vi "Test Array Data to Wave.vi"(7 "Datatype":string, 8 "error in (no error)":errorcluster, 9 "Data":variant, 10 "Dimension":string, 11 "Flag":string) -> (0 "error out":errorcluster)   [LabVIEW 2019, in "LV-Data.ITX.lvclass"]
uses:
  LV-Data.ITX.lvclass
  <vilib>/addons/_JKI Toolkits/Caraya/classes/Assert/Assert Equal Value_Variant.vi
  <vilib>/addons/_JKI Toolkits/Caraya/classes/Assert/Assert Almost Equal_Float.vi
  <vilib>/addons/_JKI Toolkits/Caraya/classes/Assert/Assert.lvclass
  <vilib>/addons/_JKI Toolkits/Caraya/classes/Test/Test.lvclass
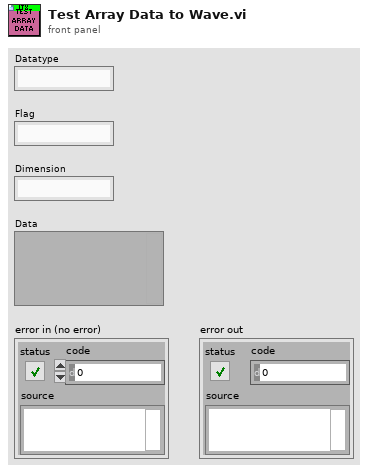
[diagram p1: front panel]
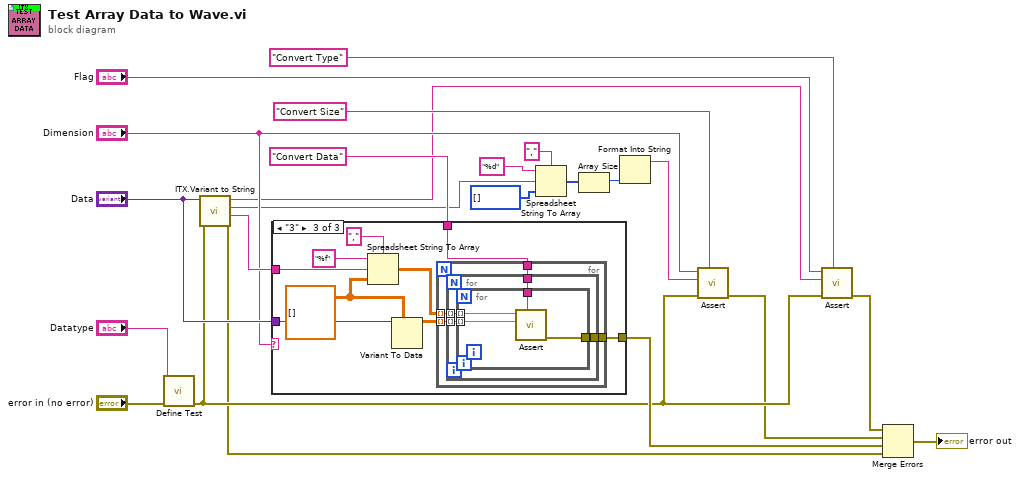
[diagram p0: block diagram]
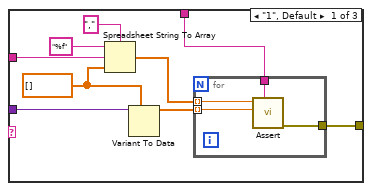
[diagram p2: hidden frame]
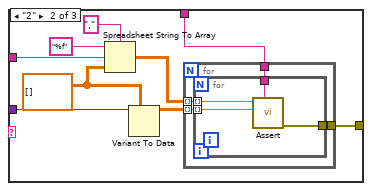
[diagram p3: hidden frame]
diagram:
  n1 = call <vilib>:"Define Test.vi"("error in (no error)"="error in (no error)", "Label (VI Title)"="Datatype") -> ("error out"=w20:errorcluster)  [unwired: 9 in]
  n2 = call "ITX.Variant to String.vi"("error in (no error)"=w20, "Data (Variant)"="Data") -> ("error out"=w18:errorcluster, "Data"=w14:string, "Size"=w3:string, "Type"=w8:string)  [unwired: 6 in]
  n3 = case shown="\"3\"" "Dimension" {
    tunnel: w14 -> [w27 w40 w57]
    tunnel: "Data" -> [w31 w44 w61]
    tunnel: [w32 w45 w62] -> w22
    tunnel: "Convert Data" ("Label") -> [w30 w43 w60]
    frame "1", Default {
      w28 = dbl[] []
      n4 = Spreadsheet String To Array(delimiter (Tab)=",", format string="%f", spreadsheet string=w27, array type (2D Dbl)=w28) -> (array=w26:dbl[])
      n5 = Variant To Data(type=w28, Variant=w31) -> (data=w29:dbl[])  [unwired: 1 in, 1 out]
      n6 = for {
        tunnel: [w36] -> w32
        tunnel: w30 -> [w35]
        tunnel: w29 -> [w34] mode=indexing
        tunnel: w26 -> [w33] mode=indexing
        n7 = call-poly <vilib>:"Assert.vi"("Label"=w35, "Y"=w34, "X"=w33) -> ("error out"=w36:errorcluster)  [unwired: 8 in]
      }
    }
    frame "2" {
      w41 = dbl[][] []
      n8 = Spreadsheet String To Array(delimiter (Tab)=",", format string="%f", spreadsheet string=w40, array type (2D Dbl)=w41) -> (array=w39:dbl[][])
      n9 = Variant To Data(type=w41, Variant=w44) -> (data=w42:dbl[][])  [unwired: 1 in, 1 out]
      n10 = for {
        tunnel: [w49] -> w45
        tunnel: w43 -> [w48]
        tunnel: w42 -> [w47] mode=indexing
        tunnel: w39 -> [w46] mode=indexing
        n11 = for {
          tunnel: [w53] -> w49
          tunnel: w48 -> [w52]
          tunnel: w47 -> [w51] mode=indexing
          tunnel: w46 -> [w50] mode=indexing
          n12 = call-poly <vilib>:"Assert.vi"("Label"=w52, "Y"=w51, "X"=w50) -> ("error out"=w53:errorcluster)  [unwired: 8 in]
        }
      }
    }
    frame "3" {
      w58 = dbl[][][] []
      n13 = Spreadsheet String To Array(delimiter (Tab)=",", format string="%f", spreadsheet string=w57, array type (2D Dbl)=w58) -> (array=w56:dbl[][][])
      n14 = Variant To Data(type=w58, Variant=w61) -> (data=w59:dbl[][][])  [unwired: 1 in, 1 out]
      n15 = for {
        tunnel: [w66] -> w62
        tunnel: w60 -> [w65]
        tunnel: w59 -> [w64] mode=indexing
        tunnel: w56 -> [w63] mode=indexing
        n16 = for {
          tunnel: [w70] -> w66
          tunnel: w65 -> [w69]
          tunnel: w64 -> [w68] mode=indexing
          tunnel: w63 -> [w67] mode=indexing
          n17 = for {
            tunnel: [w74] -> w70
            tunnel: w69 -> [w73]
            tunnel: w68 -> [w72] mode=indexing
            tunnel: w67 -> [w71] mode=indexing
            n18 = call-poly <vilib>:"Assert.vi"("Label"=w73, "Y"=w72, "X"=w71) -> ("error out"=w74:errorcluster)  [unwired: 8 in]
          }
        }
      }
    }
  }
  n19 = Spreadsheet String To Array(delimiter (Tab)=",", format string="%d", spreadsheet string=w3, array type (2D Dbl)=i32[] [] ("size(s)")) -> (array=w6:i32[])
  n20 = Array Size(array=w6) -> (size(s)=w5:i32)
  n21 = Format Into String(w5) -> (resulting string=w4:string)  [unwired: 3 in, 1 out]
  n22 = call-poly <vilib>:"Assert.vi"("Label"="Convert Size", "error in (no error)"=w20, "Y"=w4, "X"="Dimension") -> ("error out"=w16:errorcluster)  [unwired: 7 in]
  n23 = call-poly <vilib>:"Assert.vi"("Label"="Convert Type", "error in (no error)"=w20, "Y"=w8, "X"="Flag") -> ("error out"=w15:errorcluster)  [unwired: 7 in]
  n24 = Merge Errors(w15, w16, w22, w18) -> (→"error out":errorcluster)
